vi "build xml file path.vi"(8 "additional string(\"\")":string, 9 "Core":i32, 10 "Filetype":enum16{"Hardware", "Parameter"}(ring), 11 "Database Filepath in":path) -> (3 "xml path out":path)   [LabVIEW 2020]
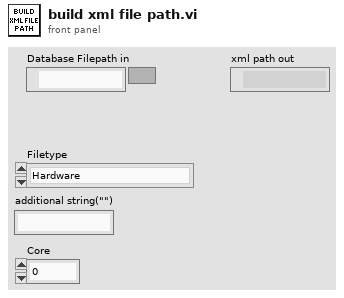
[diagram p1: front panel]
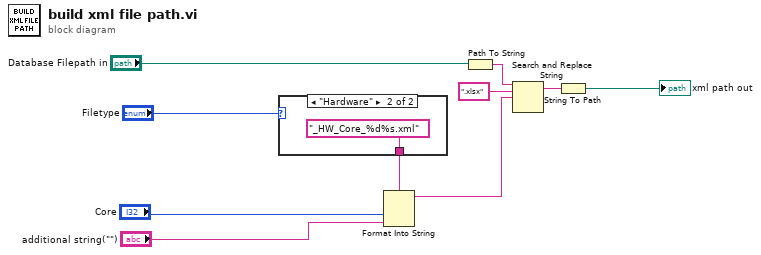
[diagram p0: block diagram]
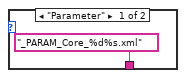
[diagram p2: hidden frame]
diagram:
  n1 = case shown="\"Hardware\"" "Filetype" {
    tunnel: ["_PARAM_Core_%d%s.xml" ("format string") "_HW_Core_%d%s.xml" ("format string")] -> w8
    frame "Parameter" {
    }
    frame "Hardware" {
    }
  }
  n2 = Format Into String(format string=w8, "Core", "additional string(\"\")") -> (resulting string=w5:string)  [unwired: 2 in, 1 out]
  n3 = Path To String(path="Database Filepath in") -> (string=w3:string)
  n4 = Search and Replace String(input string=w3, search string=".xlsx", replace string=w5) -> (result string=w9:string)  [unwired: 5 in, 3 out]
  n5 = String To Path(string=w9) -> (path=→"xml path out":path)
